vi "FPGA_I2C_I2C Port.vi"(10 "Port":u8, 11 "IO Cluster":T1={"SCK"="SCK", "DATA"="DATA"}) -> ()   [LabVIEW 2020]
doc: "Implements a single port capable of communicating with up multiple I2C slave devices."
uses:
  Controls/FPGA_I2C IO Cluster.ctl
  Controls/FPGA I2C_Port Loop State.ctl
  Controls/FPGA I2C_I2C Loop State.ctl
  <vilib>/Platform/TimedLoop/XDataNode/timing_clust.ctl
  <vilib>/Platform/TimedLoop/XDataNode/nitl_modes.ctl
  <vilib>/Platform/TimedLoop/XDataNode/wakeup.ctl
  <vilib>/rvi/Emulation/niFpgaGetClockAttributes.vi
  <vilib>/rvi/Emulation/niFpgaSctlEmulationGetInTimedLoop.vi
  <vilib>/rvi/Emulation/niFpgaEmulationReportErrorSimple.vi
  FPGA_I2C_Globals.vi
  <vilib>/rvi/Emulation/niFpgaProcessEmulError.vi
  <vilib>/rvi/Emulation/niFpgaEmulationIsFPGAContextNoSignature.vi
  <vilib>/rvi/errors/niFpgaSetErrorForExecOnDevCompSimple.vi
  <vilib>/rvi/eio/common/nirviEmuReportErrorAndStop.vi
  <vilib>/rvi/DataTransferAndStorage/Container/Common/niFpgaContainerGetUniqueNameForEmu.vi
  <vilib>/rvi/FIFO/Fifo_Resource/nirvififoEmulationSetSize.vi
  <vilib>/rvi/FIFO/Fifo_Resource/nirviFifoEmulationQueueMgr.vi
  <instcachedir>/0/nirviFifoEmulationQueueMgr_E5CAEC123FF24DC58D834DCA3CDAA9B5.lvgen/nirviFifoEmulationQueueMgr_E5CAEC123FF24DC58D834DCA3CDAA9B5_001.vi
  <vilib>/Utility/error.llb/Clear Errors.vi
  <vilib>/rvi/FIFO/Fifo_Resource/nirvififoEmulationCreateLock.vi
  <vilib>/rvi/FIFO/Fifo_Resource/nirvififoEmulationObtainLock.vi
  <vilib>/rvi/FIFO/Fifo_Resource/nirvififoEmulationReleaseLock.vi
  <vilib>/rvi/occurrence/nirviWaitOnOccurrenceBase.vi
  <vilib>/rvi/errors/nirviReportUnexpectedCaseInternalError.vi
  <vilib>/rvi/errors/nirviReportUnexpectedCaseInternalError (U32).vi
  <vilib>/rvi/FIFO/Fifo_Resource/nirvififoEmulationDetermineInputValidOut.vi
  <vilib>/rvi/Emulation/niFpgaCriticalErrorInLSC.vi
  <vilib>/rvi/eio/common/nirviEmuTemplateMethod_errors.vi
  <vilib>/rvi/DataTransferAndStorage/Container/Common/niFpgaContainerSetEmuInfo.vi
  <vilib>/rvi/DataTransferAndStorage/Container/XNode/niFpgaContainer.xnode
  <vilib>/rvi/FIFO/Fifo_Resource/nirvififoEmulationRead.vi
  <vilib>/rvi/FIFO/Fifo_Resource/nirvififoEmulationWrite.vi
  <vilib>/Platform/TimedLoop/XDataNode/XDataNode.xnode
  <vilib>/eio/EIOMethodNode/EIOMethodNode.xnode
  <vilib>/rvi/LocalResourceManager/LocalResourceManager.xnode
  <vilib>/Platform/TimedLoop/XDataNode/XDNodeRunTimeDep.lvlib
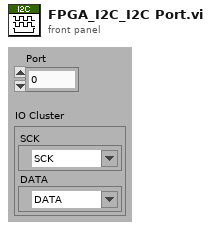
[diagram p1: front panel]
types:
  T1 = typedef "FPGA_I2C IO Cluster.ctl" = cluster{"SCK":refnum<k21>, "DATA":refnum<k21>}
  T2 = typedef "FPGA I2C_Port Loop State.ctl" = enum8{"Idle", "Start", "Configure Hardware", "Start Hardware", "Set Done", "Wait Until Done"}
  T3 = cluster{"Remaining Writes":u16, "Remaining Reads":u16, "Read New Byte":bool}
  T4 = typedef "FPGA I2C_I2C Loop State.ctl" = enum16{"Initialize", "Start Transmission", "Address/Cmd", "Write Data Byte", "Read Data Byte", "Stop Transmission"}
  T5 = typedef "XDNodeRunTimeDep.lvlib/timing_clust.ctl" = cluster{"Expected End [f-1]":u64, "Actual End [f-1]":u64, "Finished Late? [f-1]":bool, "Expected End [i-1]":u64, "Actual End [i-1]":u64, "Finished Late? [i-1]":bool, "Expected Start [i]":u64, "Actual Start [i]":u64, "Expected Start [f]":u64, "Actual Start [f]":u64, "Source Name":string, "Structure Name":string, "Period":i64, "Deadline":i64, "Offset":i64, "Start":i64, "Priority":i32, "Timeout":i32, "Mode":T6, "Wakeup Reason":T7, "Error":errorcluster, "Source Type":string, "Secondary Source Type":string, "Global End Time":u64, "Global Start Time":u64, "Frame Duration":u64, "Iteration Duration":u64, "Assigned CPU":i32, "I/O Scan Engine Mode":u32}
  T6 = typedef "XDNodeRunTimeDep.lvlib/nitl_modes.ctl" = enum32{"No Change", "Process missed periods, maintain original phase", "Discard missed periods, maintain original phase", "Process missed periods, ignore original phase", "Discard missed periods, ignore original phase"}
  T7 = typedef "XDNodeRunTimeDep.lvlib/wakeup.ctl" = enum32{"Normal", "Aborted", "Asynchronous wakeup", "Timing source error", "Timed loop error", "Timeout"}
  T8 = typedef "FPGA I2C_Cmd.ctl" = enum8{"Idle", "Write I2C", "Read I2C", "Write & Read I2C", "Configure"}
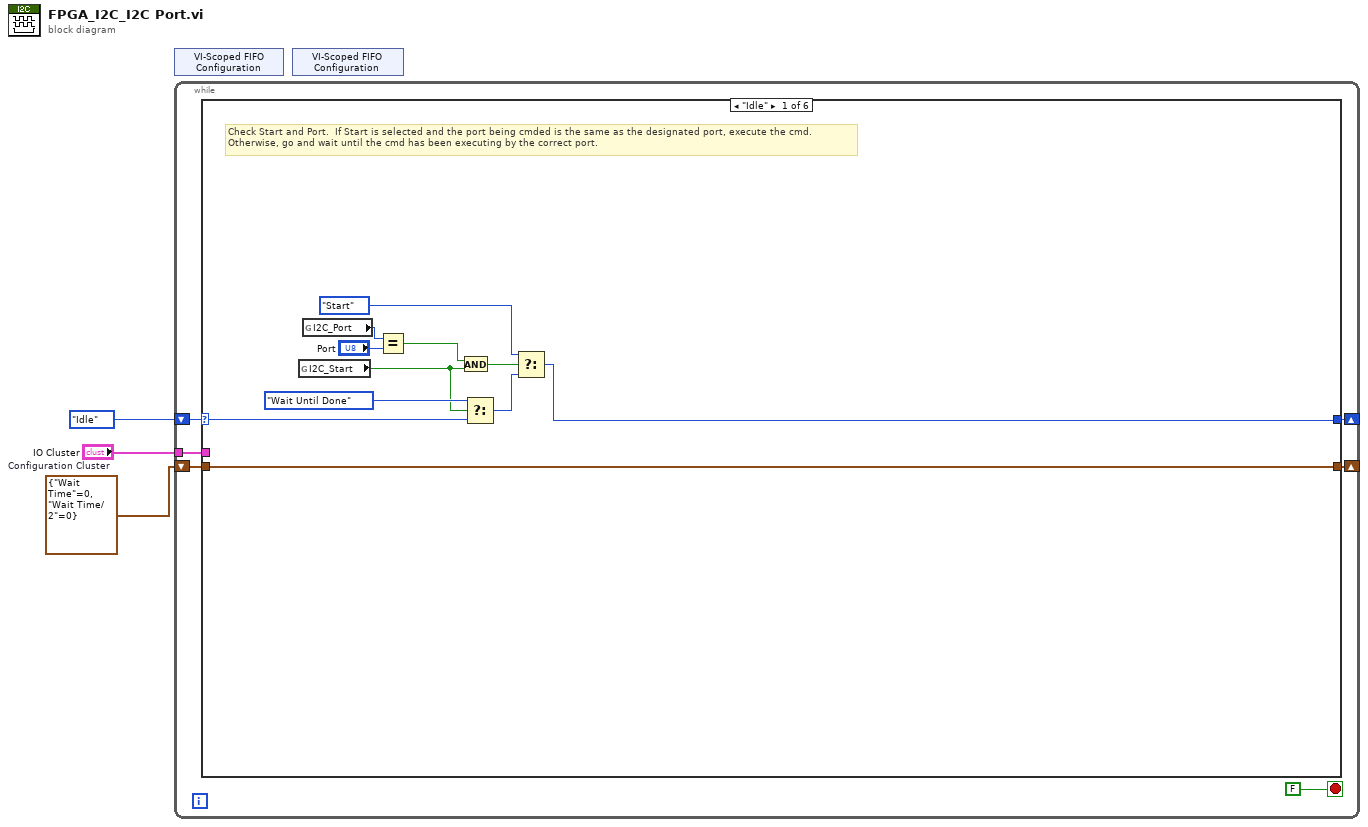
[diagram p0: block diagram]
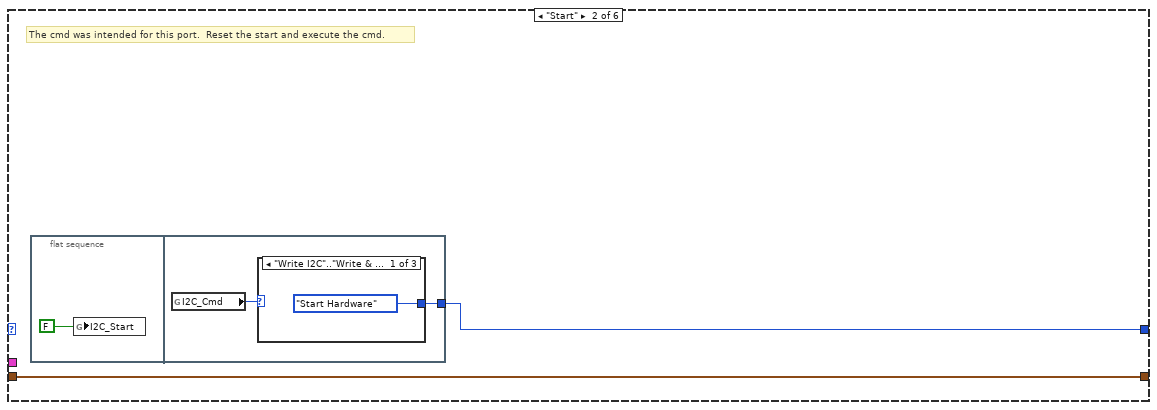
[diagram p2: hidden frame]
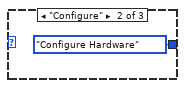
[diagram p3: hidden frame]
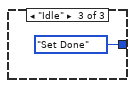
[diagram p4: hidden frame]
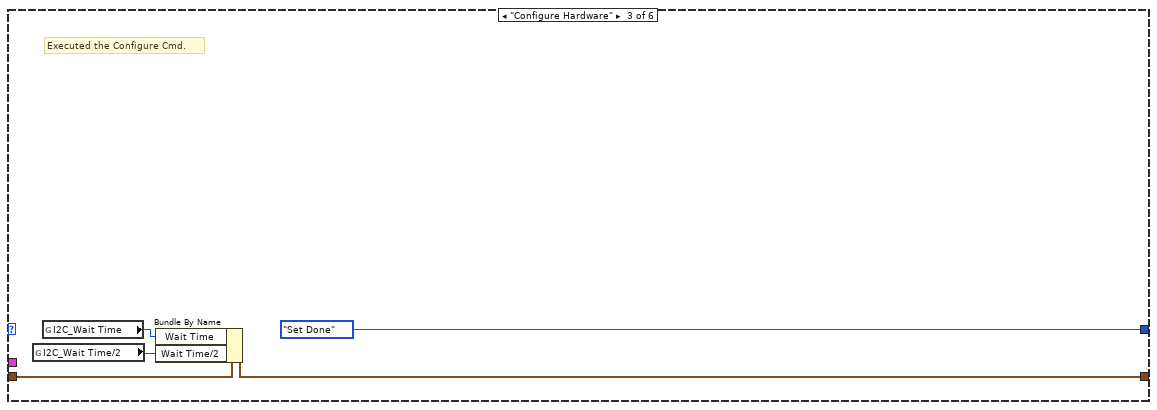
[diagram p5: hidden frame]
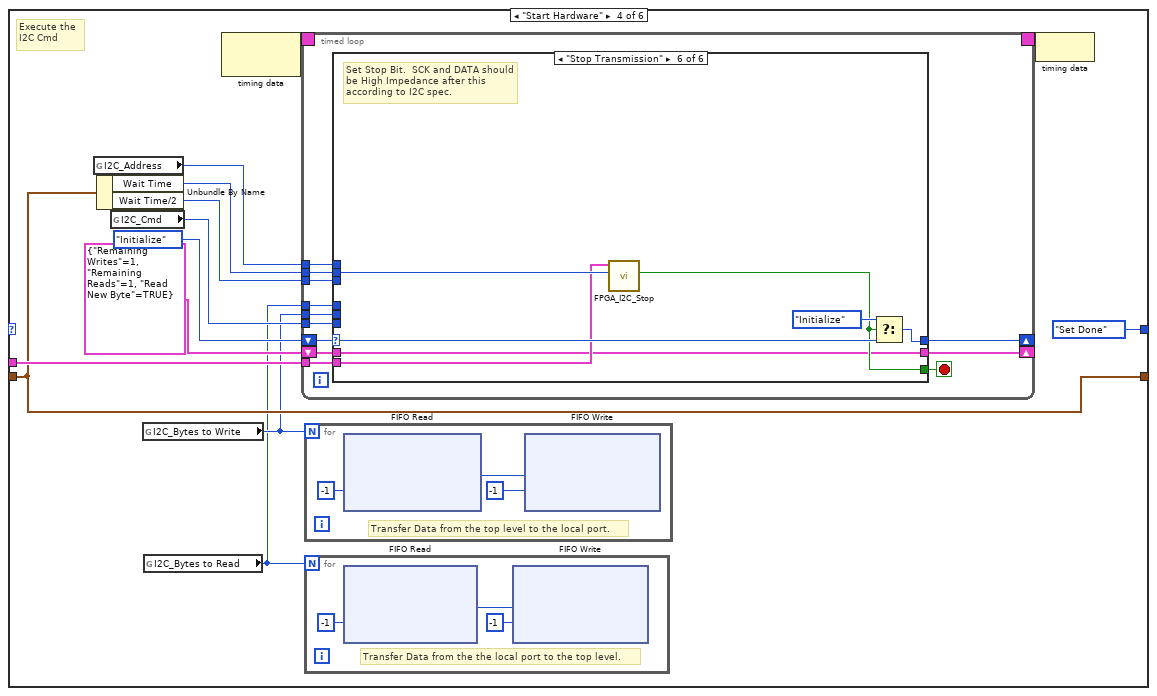
[diagram p6: hidden frame]
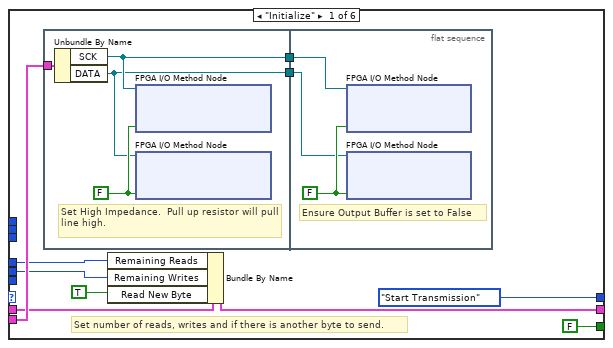
[diagram p7: hidden frame]
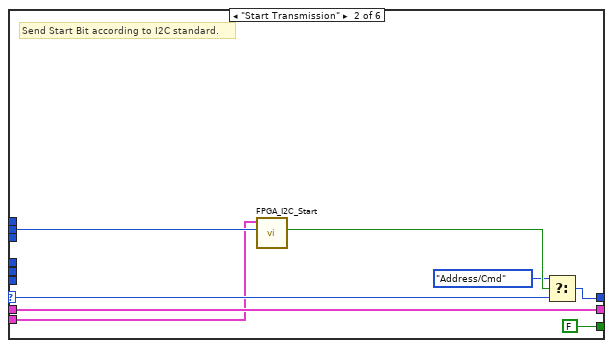
[diagram p8: hidden frame]
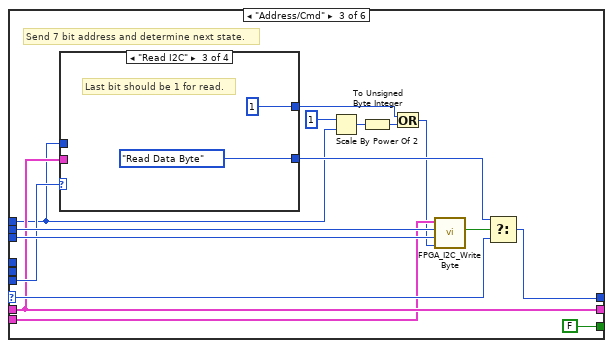
[diagram p9: hidden frame]
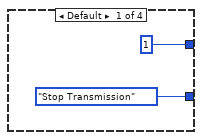
[diagram p10: hidden frame]
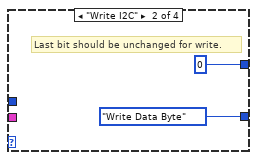
[diagram p11: hidden frame]
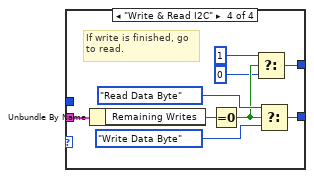
[diagram p12: hidden frame]
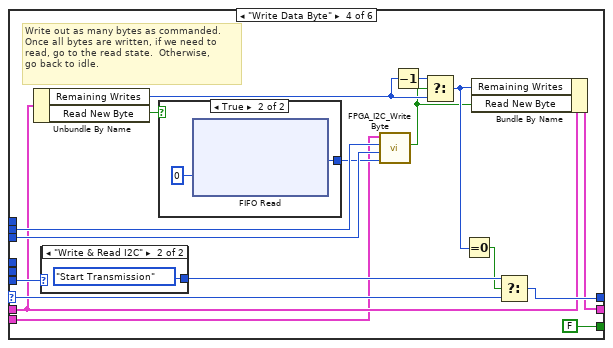
[diagram p13: hidden frame]
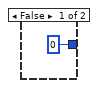
[diagram p14: hidden frame]
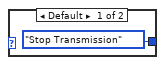
[diagram p15: hidden frame]
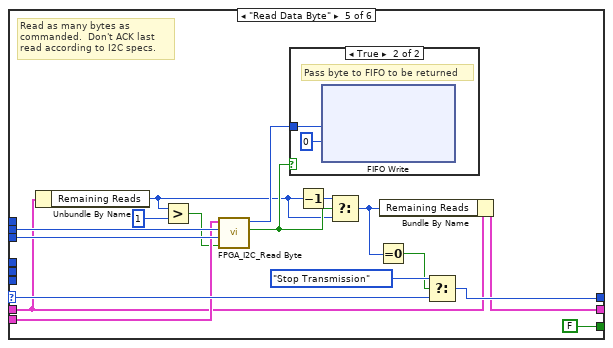
[diagram p16: hidden frame]
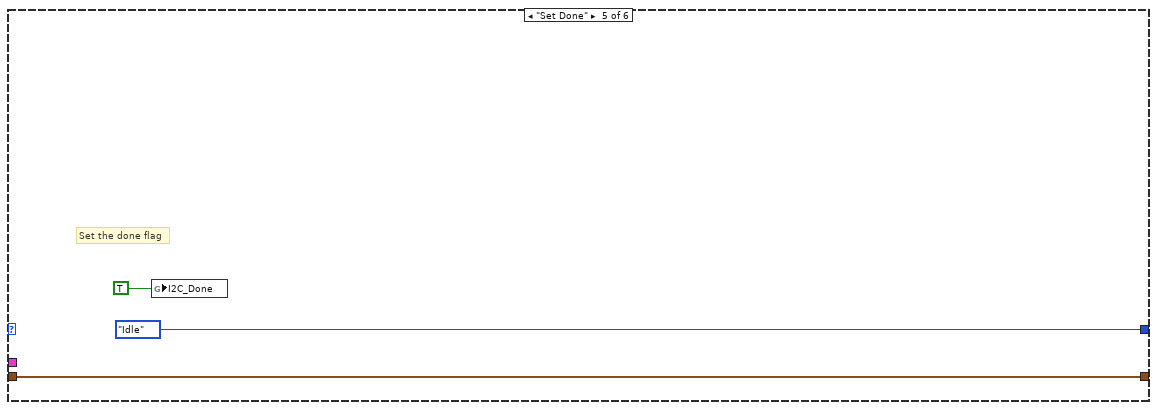
[diagram p18: hidden frame]
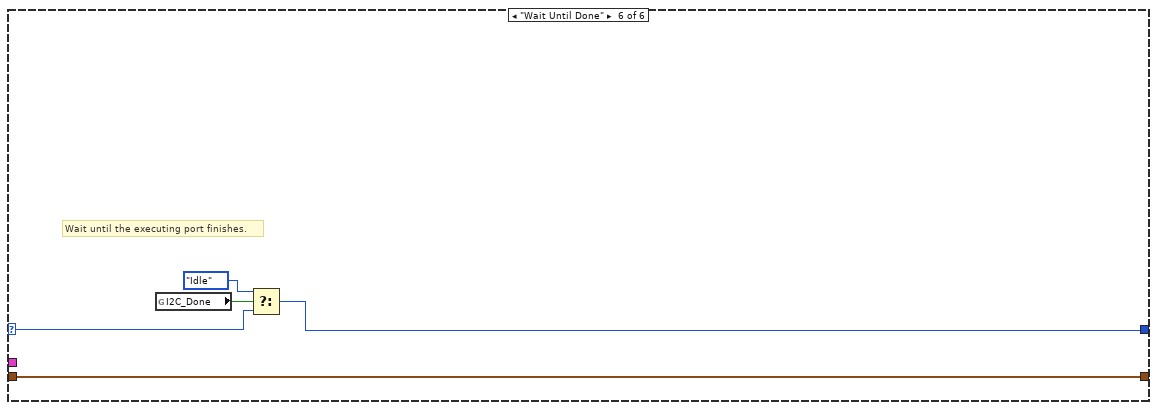
[diagram p19: hidden frame]
diagram:
  w1 = cluster{"Wait Time":u32, "Wait Time/2":u32} {"Wait Time"=0, "Wait Time/2"=0}  # Configuration Cluster
  n1 = xnode "VI-Scoped FIFO Configuration"() -> ()  [unwired: 1 out]
  n2 = while {
    shift-right: [w8] -> _
    shift-left: FPGA_I2C_Port_Loop_State."Idle" ("Action") -> [w7]
    shift-right: [w4] -> _
    shift-left: w1 -> [w6]
    tunnel: "IO Cluster" -> [w5]
    stop <- FALSE stop-if-true
    n3 = case shown="\"Idle\"" w7 {
      selector: w7 -> [w12 _ _ _ _ w179]
      tunnel: [w19 w22 FPGA_I2C_Port_Loop_State."Set Done" ("Action") FPGA_I2C_Port_Loop_State."Set Done" ("Action") FPGA_I2C_Port_Loop_State."Idle" ("Action") w178] -> w8
      tunnel: w6 -> [w15 w21 w33 w39 w174 w177]
      tunnel: w5 -> [_ _ _ w42 _ _]
      tunnel: [w15 w21 w32 w39 w174 w177] -> w4
      frame "Idle" {
        # "Check Start and Port.  If Start is selected and the port being cmded is the same as the designated port, execute the cmd.\nOtherwise, go and wait until the cmd has been executing by the correct port."
        n4 = global read "FPGA_I2C_Globals.vi" "I2C_Start"() -> (w11:bool)
        n5 = global read "FPGA_I2C_Globals.vi" "I2C_Port"() -> (w10:u8)
        n6 = Equal?(x=w10, y="Port") -> (x = y?=w13:bool)
        n7 = And(x=w13, y=w11) -> (x .and. y?=w17:bool)
        n8 = Select(t=FPGA_I2C_Port_Loop_State."Wait Until Done" ("Action"), s=w11, f=w12) -> (s? t:f=w16:T2)
        n9 = Select(t=FPGA_I2C_Port_Loop_State."Start" ("Action"), s=w17, f=w16) -> (s? t:f=w19:T2)
      }
      frame "Start" {
        # "The cmd was intended for this port.  Reset the start and execute the cmd."
        n10 = flat-sequence {
          tunnel: [w25] -> w22
          frame #0 {
            n11 = global write "FPGA_I2C_Globals.vi" "I2C_Start"(FALSE ("Write Flag")) -> ()
          }
          frame #1 {
            n12 = global read "FPGA_I2C_Globals.vi" "I2C_Cmd"() -> (w24:T8)
            n13 = case shown="\"Write I2C\"..\"Write & Read I2C\"" w24 {
              tunnel: [FPGA_I2C_Port_Loop_State."Start Hardware" ("Action") FPGA_I2C_Port_Loop_State."Configure Hardware" ("Action") FPGA_I2C_Port_Loop_State."Set Done" ("Action")] -> w25
              frame "Write I2C".."Write & Read I2C" {
              }
              frame "Configure" {
              }
              frame "Idle" {
              }
            }
          }
        }
      }
      frame "Configure Hardware" {
        # "Executed the Configure Cmd."
        n14 = global read "FPGA_I2C_Globals.vi" "I2C_Wait Time/2"() -> (w30:u32)
        n15 = global read "FPGA_I2C_Globals.vi" "I2C_Wait Time"() -> (w29:u32)
        n16 = Bundle By Name(cluster=w33, "Wait Time"=w29, "Wait Time/2"=w30) -> (w32:cluster{"Wait Time":u32, "Wait Time/2":u32})
      }
      frame "Start Hardware" {
        # "Execute the \nI2C Cmd"
        n17 = global read "FPGA_I2C_Globals.vi" "I2C_Address"() -> (w38:u16)
        n18 = Unbundle By Name(w39) -> ("Wait Time"=w41:u32, "Wait Time/2"=w40:u32)
        n19 = global read "FPGA_I2C_Globals.vi" "I2C_Cmd"() -> (w37:T8)
        n20 = global read "FPGA_I2C_Globals.vi" "I2C_Bytes to Write"() -> (w35:u16)
        n21 = global read "FPGA_I2C_Globals.vi" "I2C_Bytes to Read"() -> (w34:u16)
        n22 = node-c288() -> (w45:T5)  [unwired: 1 out]
        n23 = timed-loop {
          shift-right: [w57] -> _
          shift-left: FPGA_I2C_I2C_Loop_State."Initialize" ("Enum") -> [w58]
          timing: w45 -> [_]
          timing-out: [_] -> w44
          tunnel: w41 -> [w56]
          tunnel: w40 -> [w55]
          tunnel: w42 -> [w54]
          tunnel: w38 -> [w53]
          tunnel: w37 -> [w52]
          shift-right: [w47] -> _
          shift-left: T3 {"Remaining Writes"=1, "Remaining Reads"=1, "Read New Byte"=TRUE} -> [w50]
          tunnel: w35 -> [w49]
          tunnel: w34 -> [w48]
          stop <- w51 stop-if-true
          n24 = case shown="\"Stop Transmission\"" w58 {
            selector: w58 -> [_ w82 w99 w131 w151 w162]
            tunnel: [FPGA_I2C_I2C_Loop_State."Start Transmission" ("Enum") w80 w97 w129 w152 w160] -> w57
            tunnel: w56 -> [_ w79 w96 w128 w150 w159]
            tunnel: w55 -> [_ _ w95 w127 w149 _]
            tunnel: w54 -> [w67 w76 w86 w116 w148 w158]
            tunnel: w53 -> [_ _ w89 _ _ _]
            tunnel: w52 -> [_ _ w94 w126 _ _]
            tunnel: [FALSE FALSE FALSE FALSE FALSE w157] -> w51
            tunnel: w50 -> [w64 w78 w93 w122 w143 w156]
            tunnel: w49 -> [w61 _ _ _ _ _]
            tunnel: w48 -> [w60 _ _ _ _ _]
            tunnel: [w62 w78 w93 w120 w141 w156] -> w47
            frame "Initialize" {
              # "Set number of reads, writes and if there is another byte to send."
              n25 = flat-sequence {
                tunnel: w67 -> [w71]
                tunnel: [w70] -> w66
                tunnel: [w69] -> w65
                tunnel: w66 -> [w74]
                tunnel: w65 -> [w73]
                frame #0 {
                  w72 = FALSE ("Enable")
                  # "Set High Impedance.  Pull up resistor will pull line high."
                  n26 = Unbundle By Name(w71) -> ("SCK"=w70:refnum<k21>, "DATA"=w69:refnum<k21>)
                  n27 = xnode "FPGA I/O Method Node"("FPGA I/O In"=w70, "Enable"=w72) -> ()  [unwired: 1 out]
                  n28 = xnode "FPGA I/O Method Node"("FPGA I/O In"=w69, "Enable"=w72) -> ()  [unwired: 1 out]
                }
                frame #1 {
                  w75 = FALSE ("Enable")
                  # "Ensure Output Buffer is set to False"
                  n29 = xnode "FPGA I/O Method Node"("FPGA I/O In"=w74, "Data"=w75) -> ()  [unwired: 1 out]
                  n30 = xnode "FPGA I/O Method Node"("FPGA I/O In"=w73, "Data"=w75) -> ()  [unwired: 1 out]
                }
              }
              n31 = Bundle By Name(cluster=w64, "Remaining Reads"=w60, "Remaining Writes"=w61, "Read New Byte"=TRUE) -> (w62:T3)
            }
            frame "Start Transmission" {
              # "Send Start Bit according to I2C standard."
              n32 = call "FPGA_I2C_Start.vi"("Wait Time"=w79, "IO Cluster"=w76) -> ("Done?"=w83:bool)  [unwired: 9 out]
              n33 = Select(t=FPGA_I2C_I2C_Loop_State."Address/Cmd" ("Enum"), s=w83, f=w82) -> (s? t:f=w80:T4)
            }
            frame "Address/Cmd" {
              # "Send 7 bit address and determine next state."
              n34 = case shown="\"Read I2C\"" w94 {
                tunnel: [FPGA_I2C_I2C_Loop_State."Stop Transmission" ("Enum") FPGA_I2C_I2C_Loop_State."Write Data Byte" ("Enum") FPGA_I2C_I2C_Loop_State."Read Data Byte" ("Enum") w110] -> w98
                tunnel: w93 -> [_ _ _ w114]
                tunnel: [u8 1 u8 0 u8 1 w108] -> w90
                tunnel: w89 -> [_ _ _ _]
                frame Default {
                }
                frame "Write I2C" {
                  # "Last bit should be unchanged for write."
                }
                frame "Read I2C" {
                  # "Last bit should be 1 for read."
                }
                frame "Write & Read I2C" {
                  # "If write is finished, go\nto read."
                  n35 = Unbundle By Name(w114) -> ("Remaining Writes"=w113:u16)
                  n36 = Equal To 0?(x=w113) -> (x = 0?=w109:bool)
                  n37 = Select(t=u8 1, s=w109, f=u8 0) -> (s? t:f=w108:u8)
                  n38 = Select(t=FPGA_I2C_I2C_Loop_State."Read Data Byte" ("Enum"), s=w109, f=FPGA_I2C_I2C_Loop_State."Write Data Byte" ("Enum")) -> (s? t:f=w110:T4)
                }
              }
              n39 = Scale By Power Of 2(n=u8 1 ("y"), x=w89) -> (x*2^n=w91:u16)
              n40 = To Unsigned Byte Integer(number=w91) -> (unsigned 8bit integer=w87:u8)
              n41 = Or(x=w90, y=w87) -> (x .or. y?=w85:u8)
              n42 = call "FPGA_I2C_Write Byte.vi"("Data"=w85, "Wait Time/2"=w95, "Wait Time"=w96, "IO Cluster"=w86) -> ("Done?"=w84:bool)  [unwired: 7 out]
              n43 = Select(t=w98, s=w84, f=w99) -> (s? t:f=w97:T4)
            }
            frame "Write Data Byte" {
              # "Write out as many bytes as commanded.\nOnce all bytes are written, if we need to\nread, go to the read state.  Otherwise,\ngo back to idle."
              n44 = Unbundle By Name(w122) -> ("Remaining Writes"=w119:u16, "Read New Byte"=w125:bool)
              n45 = case shown="\"Write & Read I2C\"" w126 {
                tunnel: [FPGA_I2C_I2C_Loop_State."Stop Transmission" ("t") FPGA_I2C_I2C_Loop_State."Start Transmission" ("t")] -> w130
                frame Default {
                }
                frame "Write & Read I2C" {
                }
              }
              n46 = case shown="True" w125 {
                tunnel: [u8 0 ("Element") w133] -> w117
                frame False {
                }
                frame True {
                  n47 = xnode ("FIFO Read")("Timeout"=0) -> ("Element"=w133:u8)  [unwired: 1 in, 2 out]
                }
              }
              n48 = call "FPGA_I2C_Write Byte.vi"("Data"=w117, "Wait Time/2"=w127, "Wait Time"=w128, "IO Cluster"=w116) -> ("Done?"=w115:bool)  [unwired: 7 out]
              n49 = Decrement(x=w119) -> (x-1=w124:u16)
              n50 = Select(t=w124, s=w115, f=w119) -> (s? t:f=w121:u16)
              n51 = Equal To 0?(x=w121) -> (x = 0?=w123:bool)
              n52 = Bundle By Name(cluster=w122, "Remaining Writes"=w121, "Read New Byte"=w115) -> (w120:T3)
              n53 = Select(t=w130, s=w123, f=w131) -> (s? t:f=w129:T4)
            }
            frame "Read Data Byte" {
              # "Read as many bytes as commanded.  Don't ACK last read according to I2C specs."
              n54 = Unbundle By Name(w143) -> ("Remaining Reads"=w139:u16)
              n55 = Greater?(x=w139, y=u16 1) -> (0:w137:bool)
              n56 = call "FPGA_I2C_Read Byte.vi"("ACK?"=w137, "Wait Time/2"=w149, "Wait Time"=w150, "IO Cluster"=w148) -> ("Done?"=w144:bool, "Data"=w147:u8)  [unwired: 6 out]
              n57 = case shown="True" w144 {
                tunnel: w147 -> [_ w155]
                frame False {
                }
                frame True {
                  # "Pass byte to FIFO to be returned"
                  n58 = xnode ("FIFO Write")("Element"=w155, "Timeout"=0) -> ()  [unwired: 1 in, 2 out]
                }
              }
              n59 = Decrement(x=w139) -> (x-1=w146:u16)
              n60 = Select(t=w146, s=w144, f=w139) -> (s? t:f=w142:u16)
              n61 = Equal To 0?(x=w142) -> (x = 0?=w145:bool)
              n62 = Bundle By Name(cluster=w143, "Remaining Reads"=w142) -> (w141:T3)
              n63 = Select(t=FPGA_I2C_I2C_Loop_State."Stop Transmission", s=w145, f=w151) -> (s? t:f=w152:T4)
            }
            frame "Stop Transmission" {
              # "Set Stop Bit.  SCK and DATA should be High Impedance after this according to I2C spec."
              n64 = call "FPGA_I2C_Stop.vi"("Wait Time"=w159, "IO Cluster"=w158) -> ("Done?"=w157:bool)  [unwired: 9 out]
              n65 = Select(t=FPGA_I2C_I2C_Loop_State."Initialize" ("Enum"), s=w157, f=w162) -> (s? t:f=w160:T4)
            }
          }
        }
        n66 = for {
          N: w35 -> [_]
          # "Transfer Data from the top level to the local port."
          n67 = xnode ("FIFO Read")("Timeout"=-1) -> ("Element"=w171:u8)  [unwired: 1 in, 2 out]
          n68 = xnode ("FIFO Write")("Element"=w171, "Timeout"=-1) -> ()  [unwired: 1 in, 2 out]
        }
        n69 = for {
          N: w34 -> [_]
          # "Transfer Data from the the local port to the top level."
          n70 = xnode ("FIFO Read")("Timeout"=-1) -> ("Element"=w168:u8)  [unwired: 1 in, 2 out]
          n71 = xnode ("FIFO Write")("Element"=w168, "Timeout"=-1) -> ()  [unwired: 1 in, 2 out]
        }
        n72 = node-c288(w44) -> ()
      }
      frame "Set Done" {
        # "Set the done flag"
        n73 = global write "FPGA_I2C_Globals.vi" "I2C_Done"(TRUE ("Done")) -> ()
      }
      frame "Wait Until Done" {
        # "Wait until the executing port finishes."
        n74 = global read "FPGA_I2C_Globals.vi" "I2C_Done"() -> (w176:bool)
        n75 = Select(t=FPGA_I2C_Port_Loop_State."Idle" ("Action"), s=w176, f=w179) -> (s? t:f=w178:T2)
      }
    }
  }
  n76 = xnode "VI-Scoped FIFO Configuration"() -> ()  [unwired: 1 out]
